vi "clear_buffers.vi"(8 "error in (no error)":errorcluster, 11 "FPGA_AK101022Resonance in":refnum<class "FPGAWrapperAK101022Resonance.lvclass">) -> (0 "error out":errorcluster, 3 "FPGA_AK101022Resonance out":refnum<class "FPGAWrapperAK101022Resonance.lvclass">)   [LabVIEW 2010, in "FPGAWrapperAK101022Resonance.lvclass"]
uses:
  FPGAWrapperAK101022Resonance.lvclass
  class_data.vi
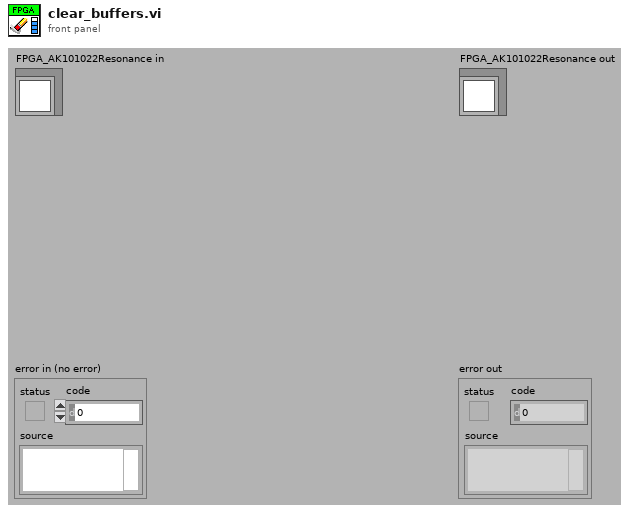
[diagram p1: front panel]
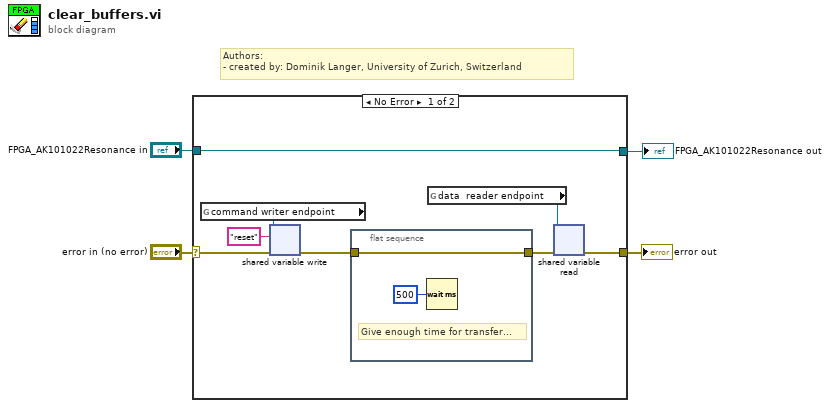
[diagram p0: block diagram]
diagram:
  # "Authors: \n- created by: Dominik Langer, University of Zurich, Switzerland"
  n1 = case shown="No Error" "error in (no error)" {
    selector: "error in (no error)" -> [w10 w16]
    tunnel: "FPGA_AK101022Resonance in" -> [w11 w15]
    tunnel: [w8 w16] -> w2
    tunnel: [w11 w15] -> w1
    frame No Error {
      n2 = global read "class_data.vi" "command writer endpoint"() -> (w12:refnum<k21>)
      n3 = shared-variable-write(w12, w10, "reset" ("data in")) -> (w6:errorcluster)  [unwired: 1 in, 2 out]
      n4 = flat-sequence {
        tunnel: w6 -> [w13]
        tunnel: [w13] -> w5
        frame #0 {
          # "Give enough time for transfer..."
          n5 = Wait (ms)(milliseconds to wait=u32 500) -> ()  [unwired: 1 out]
        }
      }
      n6 = global read "class_data.vi" "data  reader endpoint"() -> (w7:refnum<k21>)
      n7 = shared-variable-read(w7, w5) -> (w8:errorcluster)  [unwired: 2 in, 3 out]
    }
    frame Error {
    }
  }
  "error out" <- w2
  "FPGA_AK101022Resonance out" <- w1
